vi "Sensor Data (Edited).vi"() -> ()   [LabVIEW 2014]
panel:
  out "Tote too far right (inside)":bool
  out "Tote too far left (inside)":bool
  out "Tote too far right (outside)":bool
  out "Tote too far left (outside)":bool
  out "Robot Y":dbl
  out "Robot X":dbl
  out "Robot Angle":dbl
  out "Magnetometer Ang":dbl
  out "Gyro Angle":dbl
  out "Magnetic Field":cluster{"X":dbl, "Y":dbl, "Z":dbl}
  out "Back left Wheel Voltage":dbl
  out "Back Right Wheel Voltage":dbl
  out "Front Right Wheel Voltage":dbl
  out "Front Left Wheel Voltage":dbl
  out "Tote in Position/Ready to Stack":bool
  in  "Lift Encoder":dbl
  out "Wheel Distance":dbl
  in  "Lift Position 4":bool
  in  "Lift Position 3":bool
  in  "Lift Position 2":bool
  in  "Lift Position 1":bool
  in  "Lift Position 5":bool
  out "Back Left Wheel Angle":dbl
  out "Back Right Wheel Angle":dbl
  out "Front Right Wheel Angle":dbl
  out "Front Left Wheel Angle":dbl
  out "Robot Heading":dbl
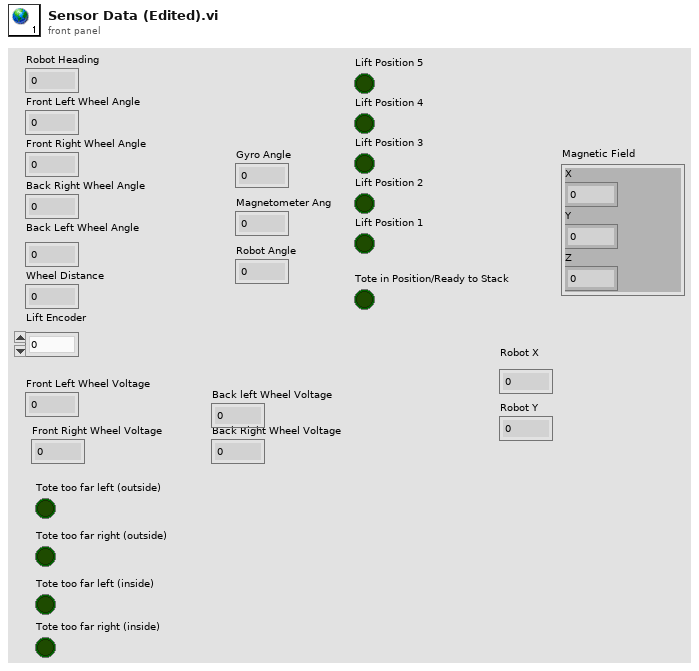
[diagram p1: front panel]
diagram:
